vi "Command Robot.vi"(11 "all rows":dbl[][](array[numeric])) -> ()   [LabVIEW 2020]
uses:
  Framework/Robot Global Data.vi
panel:
  out "X-DriveAuto":dbl
  out "Y-DriveAuto":dbl
  out "Intake Arm Down":bool
  out "Intake Arm Up":bool
  out "Intake":bool
  out "Shooter":bool
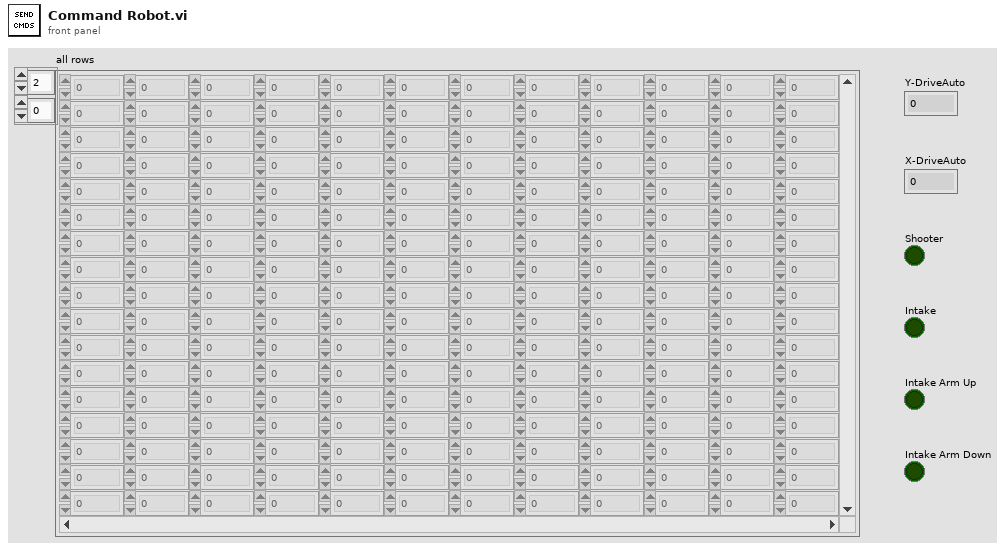
[diagram p1: front panel]
types:
  T1 = typedef "Command Status Info.ctl" = cluster{"Name":string, "Status":T2, "notifier out":T3}
  T2 = typedef "Completion Status.ctl" = enum16{"Successful", "Aborted", "Incomplete"}
  T3 = typedef "Completion Notifier.ctl" = refnum<notifier>
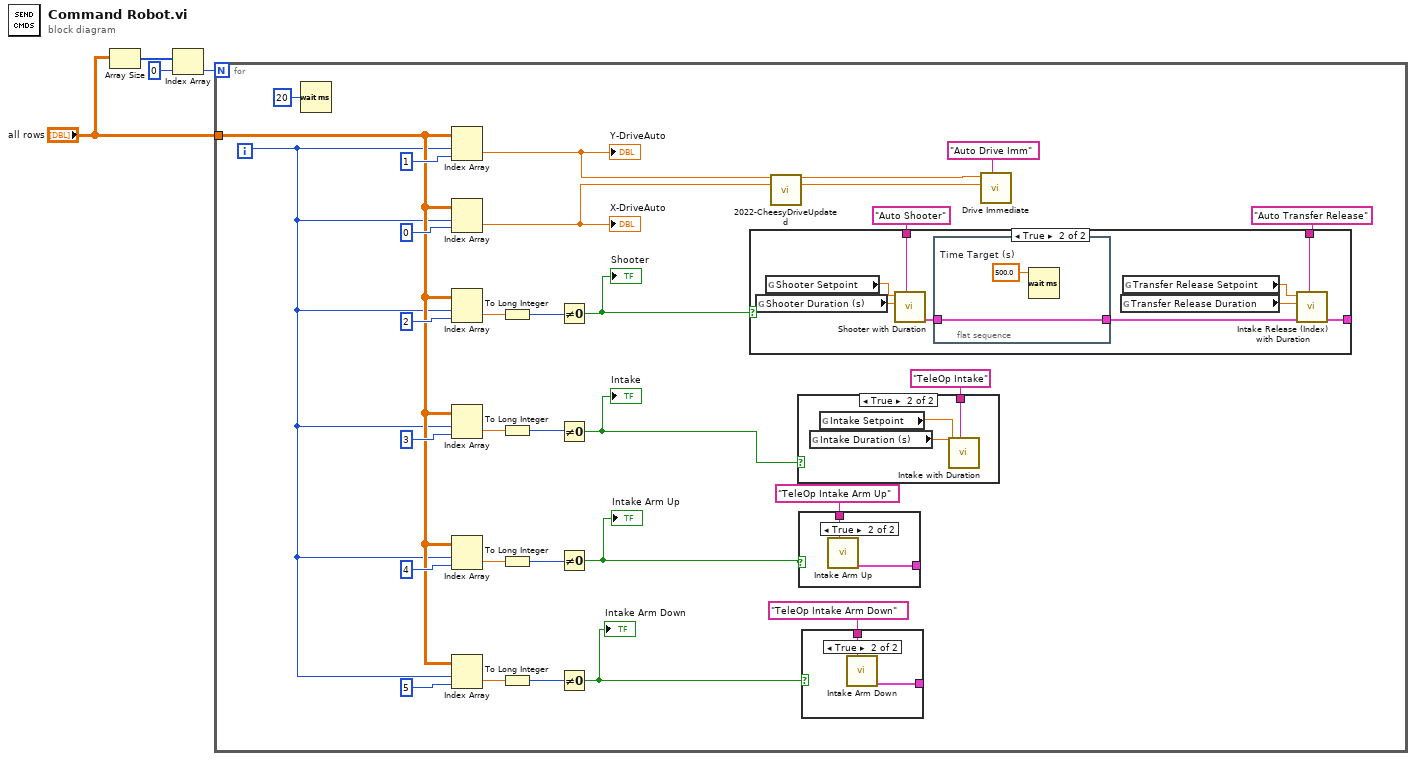
[diagram p0: block diagram]
diagram:
  n1 = Array Size(array="all rows") -> (size(s)=w2:i32[])
  n2 = Index Array(array=w2, index=0) -> (element=w1:i32)
  n3 = for {
    N: w1 -> [_]
    tunnel: "all rows" -> [w25]
    i -> [w24]
    n4 = Wait (ms)(milliseconds to wait=u32 20) -> ()  [unwired: 1 out]
    n5 = Index Array(array=w25, index (row)=w24, index (col)=1 ("disabled index (col)")) -> (element=w15:dbl)
    "Y-DriveAuto" <- w15
    n6 = Index Array(array=w25, index (row)=w24, index (col)=0 ("disabled index (col)")) -> (element=w14:dbl)
    "X-DriveAuto" <- w14
    n7 = Index Array(array=w25, index (row)=w24, index (col)=2 ("disabled index (col)")) -> (element=w29:dbl)
    n8 = Index Array(array=w25, index (row)=w24, index (col)=3 ("disabled index (col)")) -> (element=w31:dbl)
    n9 = Index Array(array=w25, index (row)=w24, index (col)=4 ("disabled index (col)")) -> (element=w33:dbl)
    n10 = Index Array(array=w25, index (row)=w24, index (col)=5 ("disabled index (col)")) -> (element=w35:dbl)
    n11 = To Long Integer(number=w29) -> (32bit integer=w23:i32)
    n12 = To Long Integer(number=w31) -> (32bit integer=w22:i32)
    n13 = To Long Integer(number=w33) -> (32bit integer=w21:i32)
    n14 = To Long Integer(number=w35) -> (32bit integer=w20:i32)
    n15 = Not Equal To 0?(x=w23) -> (x != 0?=w11:bool)
    "Shooter" <- w11
    n16 = Not Equal To 0?(x=w22) -> (x != 0?=w5:bool)
    "Intake" <- w5
    n17 = Not Equal To 0?(x=w21) -> (x != 0?=w7:bool)
    "Intake Arm Up" <- w7
    n18 = Not Equal To 0?(x=w20) -> (x != 0?=w6:bool)
    "Intake Arm Down" <- w6
    n19 = case shown="True" w11 {
      tunnel: "Auto Shooter" ("Description") -> [_ w51]
      tunnel: [_ w48] -> _
      tunnel: "Auto Transfer Release" ("Description") -> [_ w47]
      frame False {
      }
      frame True {
        n20 = global read "Robot Global Data.vi" "Shooter Duration (s)"() -> (w49:dbl)
        n21 = global read "Robot Global Data.vi" "Shooter Setpoint"() -> (w50:dbl)
        n22 = call "Shooter with Duration .vi"("Description"=w51, "Duration (s)"=w49, "Setpoint"=w50) -> ("Command Info Out"=w44:T1)  [unwired: 8 in]
        n23 = flat-sequence {
          tunnel: [w52] -> w43
          tunnel: w44 -> [w52]
          frame #0 {
            w53 = 500.0  # Time Target (s)
            n24 = Wait (ms)(milliseconds to wait=w53) -> ()  [unwired: 1 out]
          }
        }
        n25 = global read "Robot Global Data.vi" "Transfer Release Duration"() -> (w46:dbl)
        n26 = global read "Robot Global Data.vi" "Transfer Release Setpoint"() -> (w45:dbl)
        n27 = call "Intake Release (Index) with Duration.vi"("Description"=w47, "Command Info In"=w43, "Duration (s)"=w46, "Setpoint"=w45) -> ("Command Info Out"=w48:T1)  [unwired: 7 in]
      }
    }
    n28 = call "2022-CheesyDriveUpdated.vi"("Throttle"=w15, "Wheel"=w14) -> ("Left PWM"=w17:dbl, "Right PWM"=w18:dbl)  [unwired: 12 in]
    n29 = case shown="True" w5 {
      tunnel: "TeleOp Intake" ("Description") -> [_ w42]
      frame False {
      }
      frame True {
        n30 = global read "Robot Global Data.vi" "Intake Duration (s)"() -> (w40:dbl)
        n31 = global read "Robot Global Data.vi" "Intake Setpoint"() -> (w41:dbl)
        n32 = call "Intake with Duration.vi"("Description"=w42, "Duration (s)"=w40, "Setpoint"=w41) -> ()  [unwired: 8 in, 1 out]
      }
    }
    n33 = case shown="True" w7 {
      tunnel: [_ w37] -> _
      tunnel: "TeleOp Intake Arm Up" ("Description") -> [_ w36]
      frame False {
      }
      frame True {
        n34 = call "Intake Arm Up.vi"("Description"=w36) -> ("Command Info Out"=w37:T1)  [unwired: 10 in]
      }
    }
    n35 = case shown="True" w6 {
      tunnel: "TeleOp Intake Arm Down" ("Description") -> [_ w39]
      tunnel: [_ w38] -> _
      frame False {
      }
      frame True {
        n36 = call "Intake Arm Down.vi"("Description"=w39) -> ("Command Info Out"=w38:T1)  [unwired: 10 in]
      }
    }
    n37 = call "Drive Immediate.vi"("Description"="Auto Drive Imm", "Right Setpoint"=w18, "Left Setpoint"=w17) -> ()  [unwired: 8 in, 1 out]
  }
